vi "Complex Matrix Exp.vi"(3 "Input Matrix":T1) -> (0 "error":i32, 1 "Matrix Exp":T1)   [LabVIEW 2020, in "NI_AALBase.lvlib"]
doc: "Computes the exponential of a square <B>Input Matrix</B>. Wire data to the <B>Input Matrix</B> input to determine the polymorphic instance to use or manually select the instance."
uses:
  <vilib>/Analysis/NI_AALBase.lvlib
  <vilib>/Analysis/Matrix/Datatypes/ComplexMatrix.ctl
  <resource>/lvanlys.dll
  <vilib>/Analysis/Matrix/NI_Matrix.lvlib
panel:
  # "Complex Matrix Exp"
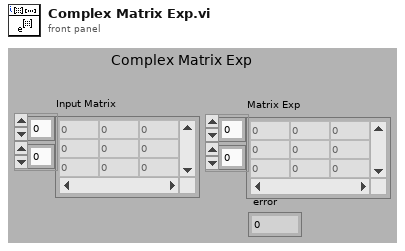
[diagram p1: front panel]
types:
  T1 = typedef "NI_Matrix.lvlib/ComplexMatrix.ctl" = cdb[][]
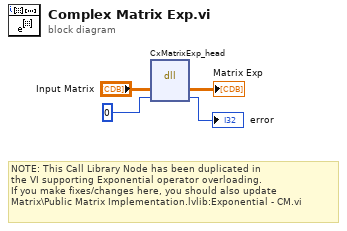
[diagram p0: block diagram]
diagram:
  # "NOTE: This Call Library Node has been duplicated in\nthe VI supporting Exponential operator overloading.\nIf you make fixes/changes here, you should also update\nMatrix\\Public Matrix Implementation.lvlib:Exponential - CM.vi"
  n1 = dll-call lib="e:/builds/penguin/labview/branches/2020/dev/dist/resource/lvanlys.*" fn="CxMatrixExp_head"("Input Matrix"="Input Matrix", 0) -> ("Input Matrix"=→"Matrix Exp":T1, →"error":i32)  [unwired: 4 in, 2 out]
